vi "ScannedImage.vi"(1 "Get/Set":bool, 2 "Scanned Image (input)":T1={"BinningMicroS"=0.0, "OverflowConstant"=0.0, "MacrotimeCycle"=0.0, "Trace"=[], "Retrace"=[], "current line"=7, "current plane"=0} {"MacrotimeCycle" format="%.2f"; "OverflowConstant" format="%.2f"; "BinningMicroS" format="%.2f"}) -> (0 "Scanned Image (output)":T1={"BinningMicroS"=0.0, "OverflowConstant"=0.0, "MacrotimeCycle"=0.0, "Trace"=[], "Retrace"=[], "current line"=7, "current plane"=0} {"MacrotimeCycle" format="%.2f"; "OverflowConstant" format="%.2f"; "BinningMicroS" format="%.2f"})   [LabVIEW 2009]
uses:
  ScannedImage.ctl
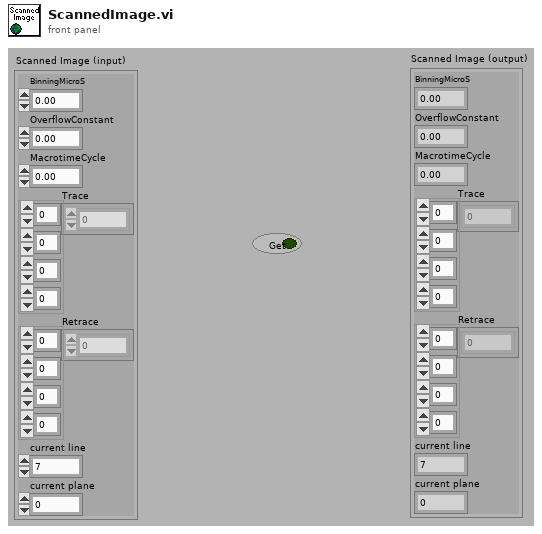
[diagram p1: front panel]
types:
  T1 = typedef "ScannedImage.ctl" = cluster{"BinningMicroS":dbl, "OverflowConstant":dbl, "MacrotimeCycle":dbl, "Trace":u32[][][][], "Retrace":u32[][][][], "current line":i32, "current plane":i32}
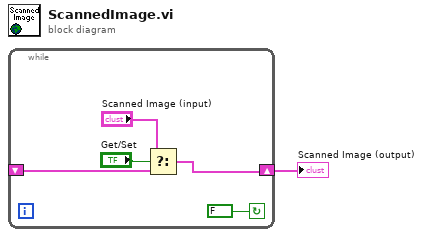
[diagram p0: block diagram]
diagram:
  n1 = while {
    shift-right: [w4] -> w1
    shift-left: _ -> [w5]
    stop <- FALSE continue-if-true
    n2 = Select(t="Scanned Image (input)", s="Get/Set", f=w5) -> (s? t:f=w4:T1)
  }
  "Scanned Image (output)" <- w1
